vi "LCR_AutoChangeUnits.vi"(4 "Secondary Ref":refnum<vi>, 5 "Secondary Unit":T1, 6 "Primary Ref":refnum<vi>, 7 "Primary Unit":T1) -> ()   [LabVIEW 2021]
uses:
  UnitEnum.ctl
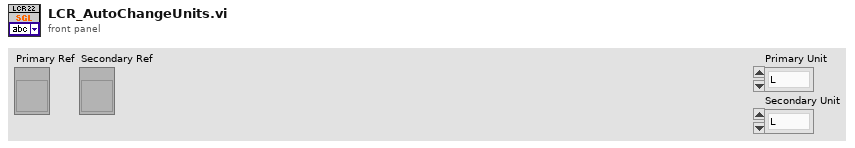
[diagram p1: front panel]
types:
  T1 = typedef "UnitEnum.ctl" = enum16{"L", "R", "C", "Z", "X", "Q", "Theta", "Y", "N", "M", "G", "B", "D"}
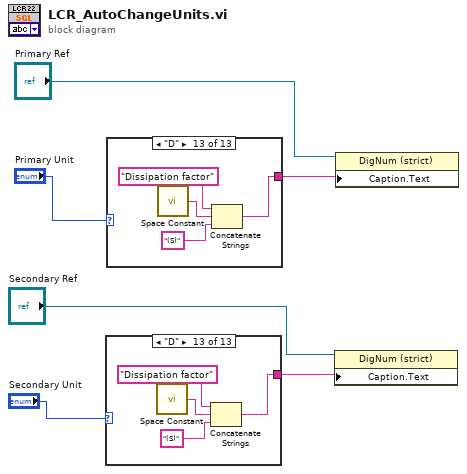
[diagram p0: block diagram]
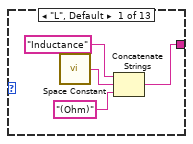
[diagram p2: hidden frame]
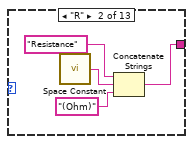
[diagram p3: hidden frame]
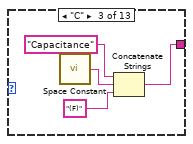
[diagram p4: hidden frame]
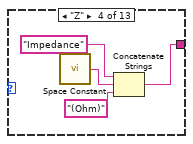
[diagram p5: hidden frame]
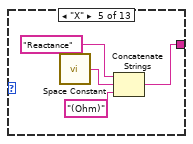
[diagram p6: hidden frame]
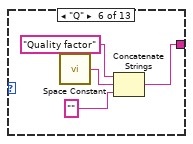
[diagram p7: hidden frame]
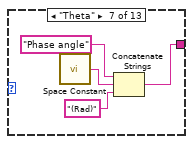
[diagram p8: hidden frame]
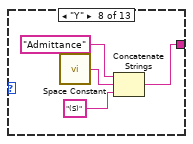
[diagram p9: hidden frame]
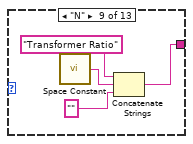
[diagram p10: hidden frame]
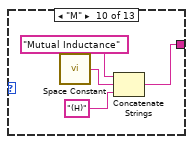
[diagram p11: hidden frame]
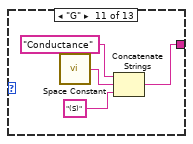
[diagram p12: hidden frame]
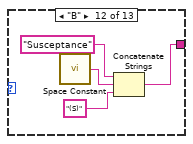
[diagram p13: hidden frame]
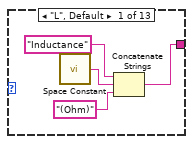
[diagram p14: hidden frame]
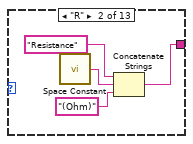
[diagram p15: hidden frame]
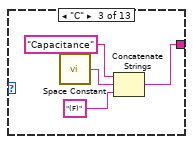
[diagram p16: hidden frame]
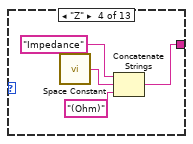
[diagram p17: hidden frame]
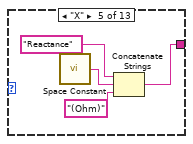
[diagram p18: hidden frame]
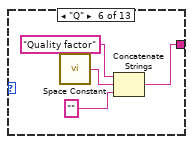
[diagram p19: hidden frame]
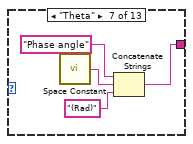
[diagram p20: hidden frame]
diagram:
  n1 = case shown="\"D\"" "Secondary Unit" {
    tunnel: [w7 w11 w15 w19 w23 w27 w31 w35 w39 w43 w47 w51 w55] -> w3
    frame "L", Default {
      n2 = call <vilib>:"Space Constant.vi"() -> ("String"=w9:string)
      n3 = Concatenate Strings("Inductance", w9, "(Ohm)") -> (w7:string)
    }
    frame "R" {
      n4 = call <vilib>:"Space Constant.vi"() -> ("String"=w13:string)
      n5 = Concatenate Strings("Resistance", w13, "(Ohm)") -> (w11:string)
    }
    frame "C" {
      n6 = call <vilib>:"Space Constant.vi"() -> ("String"=w17:string)
      n7 = Concatenate Strings("Capacitance", w17, "(F)") -> (w15:string)
    }
    frame "Z" {
      n8 = call <vilib>:"Space Constant.vi"() -> ("String"=w21:string)
      n9 = Concatenate Strings("Impedance", w21, "(Ohm)") -> (w19:string)
    }
    frame "X" {
      n10 = call <vilib>:"Space Constant.vi"() -> ("String"=w25:string)
      n11 = Concatenate Strings("Reactance", w25, "(Ohm)") -> (w23:string)
    }
    frame "Q" {
      n12 = call <vilib>:"Space Constant.vi"() -> ("String"=w29:string)
      n13 = Concatenate Strings("Quality factor", w29, "") -> (w27:string)
    }
    frame "Theta" {
      n14 = call <vilib>:"Space Constant.vi"() -> ("String"=w33:string)
      n15 = Concatenate Strings("Phase angle", w33, "(Rad)") -> (w31:string)
    }
    frame "Y" {
      n16 = call <vilib>:"Space Constant.vi"() -> ("String"=w37:string)
      n17 = Concatenate Strings("Admittance", w37, "(S)") -> (w35:string)
    }
    frame "N" {
      n18 = call <vilib>:"Space Constant.vi"() -> ("String"=w41:string)
      n19 = Concatenate Strings("Transformer Ratio", w41, "") -> (w39:string)
    }
    frame "M" {
      n20 = call <vilib>:"Space Constant.vi"() -> ("String"=w45:string)
      n21 = Concatenate Strings("Mutual Inductance", w45, "(H)") -> (w43:string)
    }
    frame "G" {
      n22 = call <vilib>:"Space Constant.vi"() -> ("String"=w49:string)
      n23 = Concatenate Strings("Conductance", w49, "(S)") -> (w47:string)
    }
    frame "B" {
      n24 = call <vilib>:"Space Constant.vi"() -> ("String"=w53:string)
      n25 = Concatenate Strings("Susceptance", w53, "(S)") -> (w51:string)
    }
    frame "D" {
      n26 = call <vilib>:"Space Constant.vi"() -> ("String"=w57:string)
      n27 = Concatenate Strings("Dissipation factor", w57, "(S)") -> (w55:string)
    }
  }
  n28 = case shown="\"D\"" "Primary Unit" {
    tunnel: [w59 w63 w67 w71 w75 w79 w83 w87 w91 w95 w99 w103 w107] -> w4
    frame "L", Default {
      n29 = call <vilib>:"Space Constant.vi"() -> ("String"=w61:string)
      n30 = Concatenate Strings("Inductance", w61, "(Ohm)") -> (w59:string)
    }
    frame "R" {
      n31 = call <vilib>:"Space Constant.vi"() -> ("String"=w65:string)
      n32 = Concatenate Strings("Resistance", w65, "(Ohm)") -> (w63:string)
    }
    frame "C" {
      n33 = call <vilib>:"Space Constant.vi"() -> ("String"=w69:string)
      n34 = Concatenate Strings("Capacitance", w69, "(F)") -> (w67:string)
    }
    frame "Z" {
      n35 = call <vilib>:"Space Constant.vi"() -> ("String"=w73:string)
      n36 = Concatenate Strings("Impedance", w73, "(Ohm)") -> (w71:string)
    }
    frame "X" {
      n37 = call <vilib>:"Space Constant.vi"() -> ("String"=w77:string)
      n38 = Concatenate Strings("Reactance", w77, "(Ohm)") -> (w75:string)
    }
    frame "Q" {
      n39 = call <vilib>:"Space Constant.vi"() -> ("String"=w81:string)
      n40 = Concatenate Strings("Quality factor", w81, "") -> (w79:string)
    }
    frame "Theta" {
      n41 = call <vilib>:"Space Constant.vi"() -> ("String"=w85:string)
      n42 = Concatenate Strings("Phase angle", w85, "(Rad)") -> (w83:string)
    }
    frame "Y" {
      n43 = call <vilib>:"Space Constant.vi"() -> ("String"=w89:string)
      n44 = Concatenate Strings("Admittance", w89, "(S)") -> (w87:string)
    }
    frame "N" {
      n45 = call <vilib>:"Space Constant.vi"() -> ("String"=w93:string)
      n46 = Concatenate Strings("Transformer Ratio", w93, "") -> (w91:string)
    }
    frame "M" {
      n47 = call <vilib>:"Space Constant.vi"() -> ("String"=w97:string)
      n48 = Concatenate Strings("Mutual Inductance", w97, "(H)") -> (w95:string)
    }
    frame "G" {
      n49 = call <vilib>:"Space Constant.vi"() -> ("String"=w101:string)
      n50 = Concatenate Strings("Conductance", w101, "(S)") -> (w99:string)
    }
    frame "B" {
      n51 = call <vilib>:"Space Constant.vi"() -> ("String"=w105:string)
      n52 = Concatenate Strings("Susceptance", w105, "(S)") -> (w103:string)
    }
    frame "D" {
      n53 = call <vilib>:"Space Constant.vi"() -> ("String"=w109:string)
      n54 = Concatenate Strings("Dissipation factor", w109, "(S)") -> (w107:string)
    }
  }
  n55 = property class="DigNum (strict)"(reference="Secondary Ref", "Caption.Text"=w3) -> ()  [unwired: 1 in, 2 out]
  n56 = property class="DigNum (strict)"(reference="Primary Ref", "Caption.Text"=w4) -> ()  [unwired: 1 in, 2 out]
